vi "test.workspace_add.vi"() -> ()   [LabVIEW 2020]
uses:
  Nominal Client.lvclass
  9ddb49fb-05ed-4eb3-8508-173ebe20c98b.vi
  730c9c5b-7bb2-47cf-818b-6e2ed47344d4.vi
  <vilib>/JDP Science/JSONtext/JSONtext.lvlib
panel:
  out "error out":errorcluster
  out "JSON payload out":string
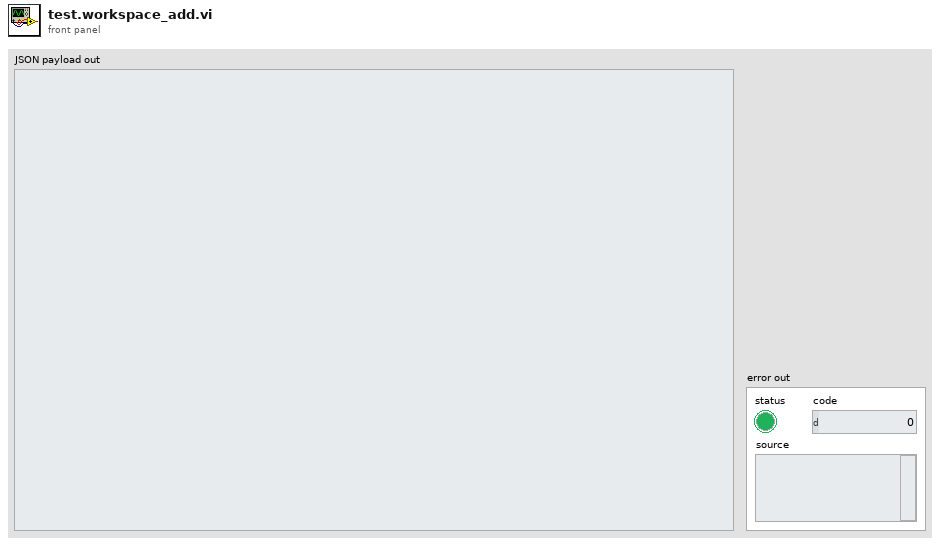
[diagram p1: front panel]
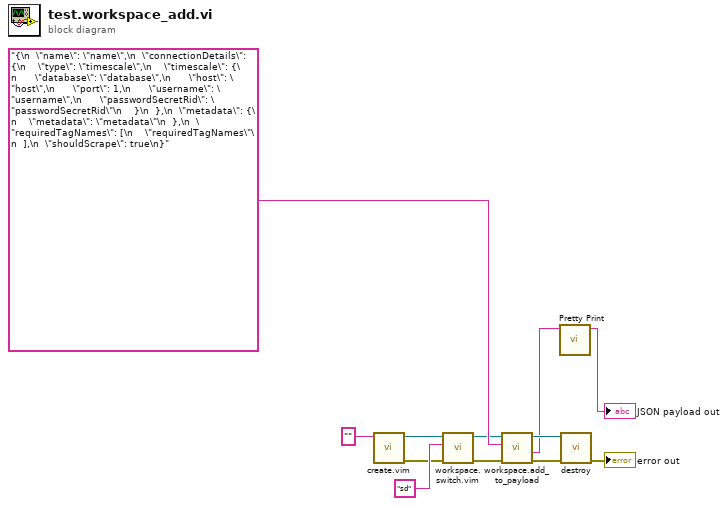
[diagram p0: block diagram]
diagram:
  n1 = call "create.vim"("API Token (string or path)"="" ("Workspace RID (string or path)")) -> ("error out"=w5:errorcluster, "Nominal Client"=w6:refnum<class "Nominal Client.lvclass">)  [unwired: 9 in]
  n2 = call "workspace.switch.vim"("error in"=w5, "Workspace RID (string or path)"="sd", "Nominal Client in"=w6) -> ("error out"=w12:errorcluster, "Nominal Client out"=w8:refnum<class "Nominal Client.lvclass">)  [unwired: 7 in]
  n3 = call "workspace.add_to_payload.vi"("error in"=w12, "JSON payload in"="{\n  \"name\": \"name\",\n  \"connectionDetails\": {\n    \"type\": \"timescale\",\n    \"timescale\": {\n      \"database\": \"database\",\n      \"host\": \"host\",\n      \"port\": 1,\n      \"username\": \"username\",\n      \"passwordSecretRid\": \"passwordSecretRid\"\n    }\n  },\n  \"metadata\": {\n    \"metadata\": \"metadata\"\n  },\n  \"requiredTagNames\": [\n    \"requiredTagNames\"\n  ],\n  \"shouldScrape\": true\n}", "Nominal Client in"=w8) -> ("error out"=w9:errorcluster, "JSON payload out"=w1:string, "Nominal Client out"=w7:refnum<class "Nominal Client.lvclass">)  [unwired: 6 in]
  n4 = call <vilib>:"Pretty Print.vi"("JSON"=w1) -> ("<JSON>"=→"JSON payload out":string)  [unwired: 8 in, 2 out]
  n5 = call "destroy.vi"("error in"=w9, "Nominal Client"=w7) -> ("error out"=→"error out":errorcluster)  [unwired: 9 in]
